vi "Enable Close Outlet.vi"(0 "FPGA API in":refnum<class "FPGA API.lvclass">, 11 "error in (no error)":errorcluster, 13 "Direction":T1=enum."Chamber") -> (4 "FPGA API out":refnum<class "FPGA API.lvclass">, 15 "error out":errorcluster)   [LabVIEW 2019, in "FPGA API.lvclass"]
uses:
  FPGA API.lvclass
  TypeDef/Direction.ctl
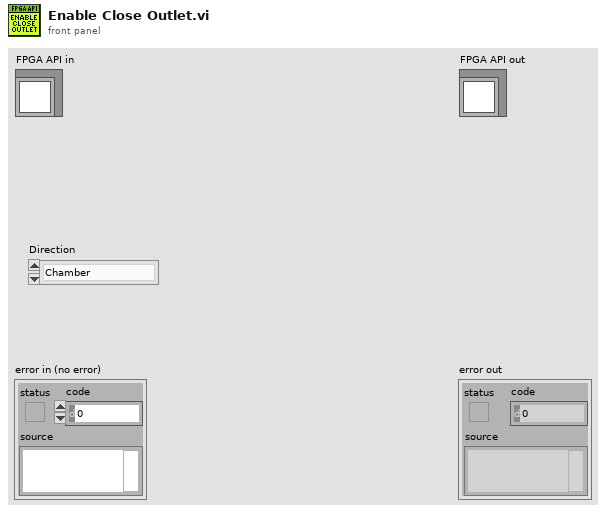
[diagram p1: front panel]
types:
  T1 = typedef "Direction.ctl" = enum16{"None", "DUT", "Chamber"}
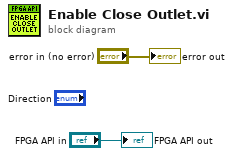
[diagram p0: block diagram]
diagram:
  "error out" <- "error in (no error)"
  "FPGA API out" <- "FPGA API in"
